vi "0x06PresetSingleRegister.vi"(6 "Data":u16, 8 "error in (no error)":errorcluster, 9 "Register":u16, 10 "Addressc":u8, 11 "ASCII in":refnum<class "ASCII.lvclass">) -> (0 "error out":errorcluster, 2 "Frame":string, 3 "ASCII out":refnum<class "ASCII.lvclass">)   [LabVIEW 2017, in "ModBUS.lvlib" / "ASCII.lvclass"]
uses:
  ASCII.lvclass
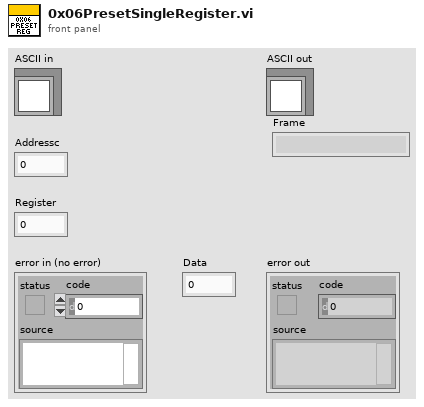
[diagram p1: front panel]
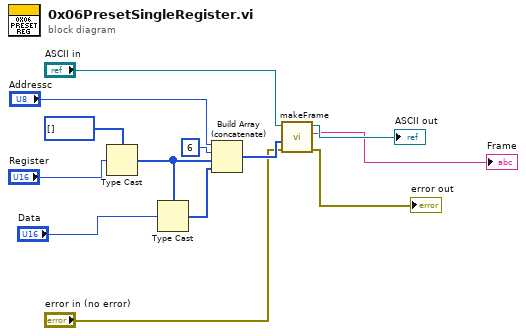
[diagram p0: block diagram]
diagram:
  n1 = Type Cast(type=u8[] [], x="Register") -> (*(type *) &x=w9:u8[])
  n2 = Type Cast(type=w9, x="Data") -> (*(type *) &x=w7:u8[])
  n3 = Build Array (concatenate)("Addressc", u8 6 ("element"), w9, w7) -> (w4:u8[])
  n4 = call-dynamic "makeFrame.vi"("error in (no error)"="error in (no error)", "Data"=w4, "ASCII in"="ASCII in") -> ("error out"=→"error out":errorcluster, "Frame"=→"Frame":string, "ASCII out"=→"ASCII out":refnum<class "ASCII.lvclass">)  [unwired: 6 in]
